vi "Object_Editor_ConfigFP.vi"(0 "reference in":refnum<class "Object_Editor.lvclass">, 5 "error in (no error)":errorcluster) -> (14 "reference out":refnum<class "Object_Editor.lvclass">, 19 "error out":errorcluster)   [LabVIEW 2022 SP3, in "Object_Editor.lvlib" / "Object_Editor.lvclass"]
uses:
  Object_Editor.lvclass
  protected/Config.ctl
  Components/ViPER.lvlibp/ViPER.lvclass
  C:/Projects/Medulla/ViPER/ViPER_ProjectTemplates/ProjectTemplates/Source/Core/ViPER/Components/ViPER.lvlibp/ViPER.lvclass
panel:
  in  "Config":T1
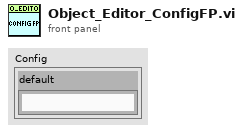
[diagram p1: front panel]
types:
  T1 = typedef "Object_Editor.lvlib/Object_Editor.lvclass/Config.ctl" = cluster{"default":string}
  T2 = enum32{"Invalid", "Standard", "Closed", "Hidden", "Minimized", "Maximized"}
  T3 = typedef "Object_Editor.lvlib/Object_Editor.lvclass/ObjectAttributes.ctl" = cluster{"Config":T1, "Tree":refnum<vi>, "Mod_Bit":bool, "File_Path":path, "Object":refnum<class "ViPER.lvclass">}
  T4 = typedef "LVRectTypeDef.ctl" = cluster{"Left":i16, "Top":i16, "Right":i16, "Bottom":i16}
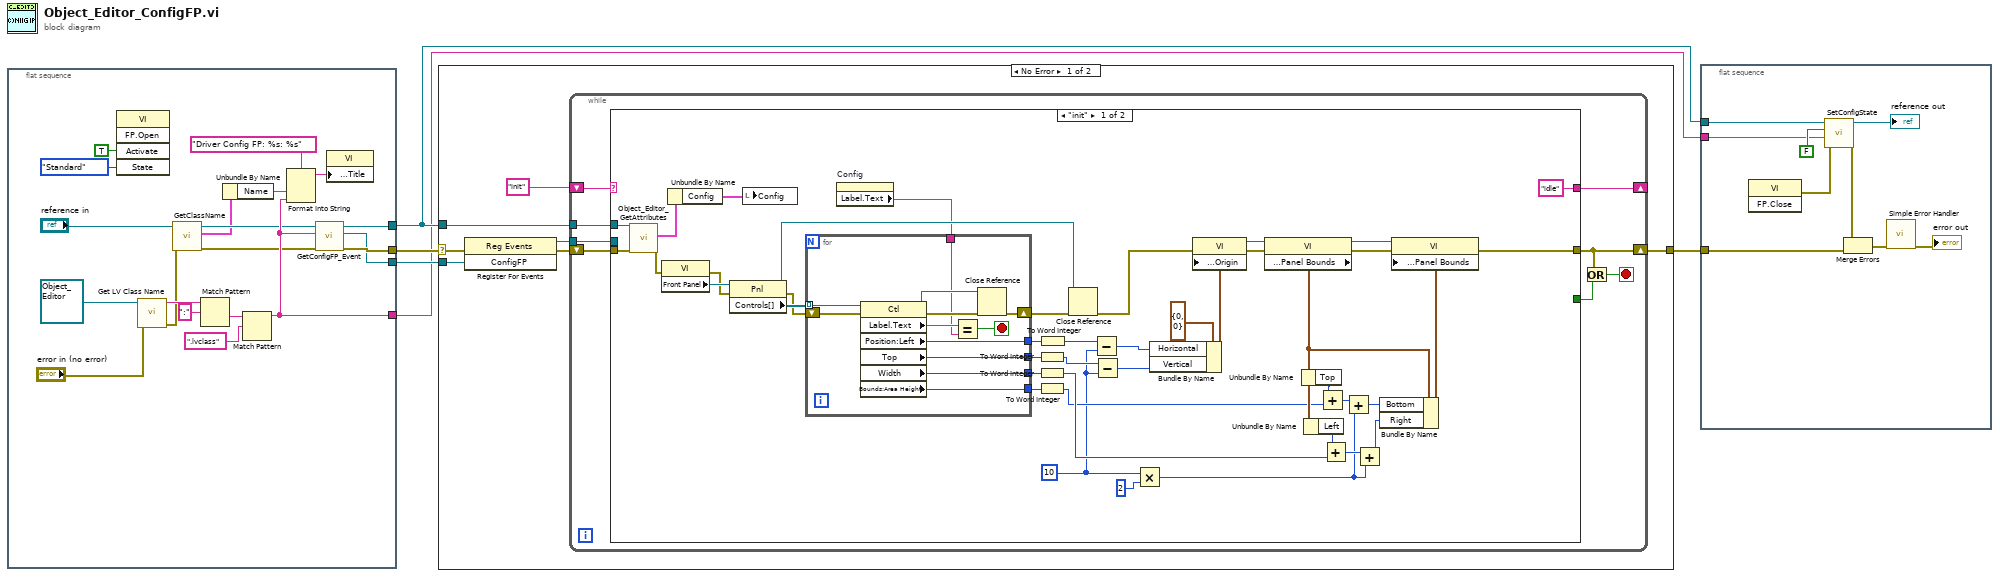
[diagram p0: block diagram]
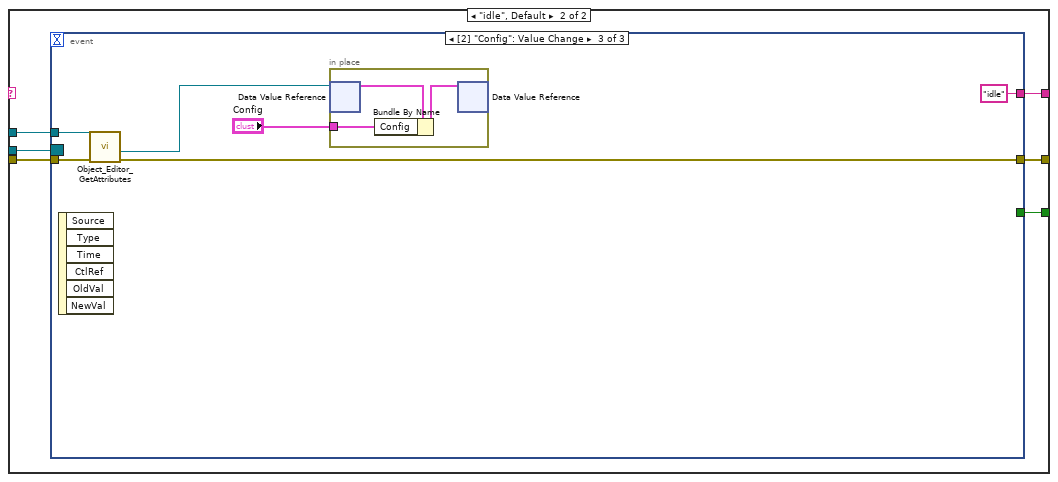
[diagram p2: hidden frame]
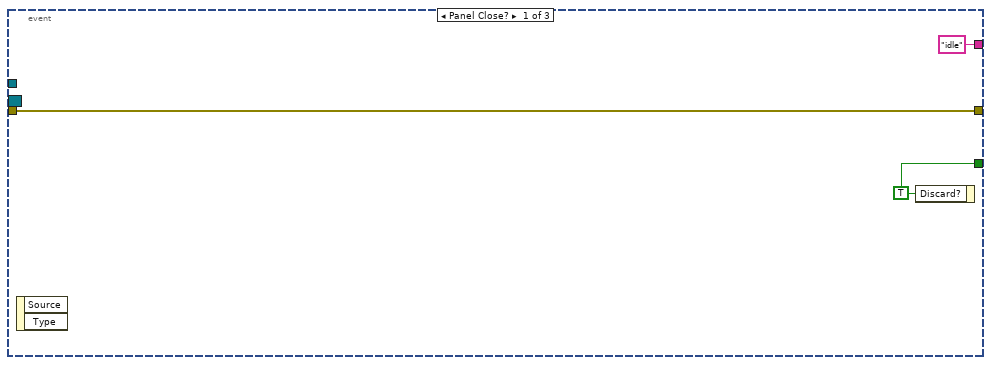
[diagram p3: hidden frame]
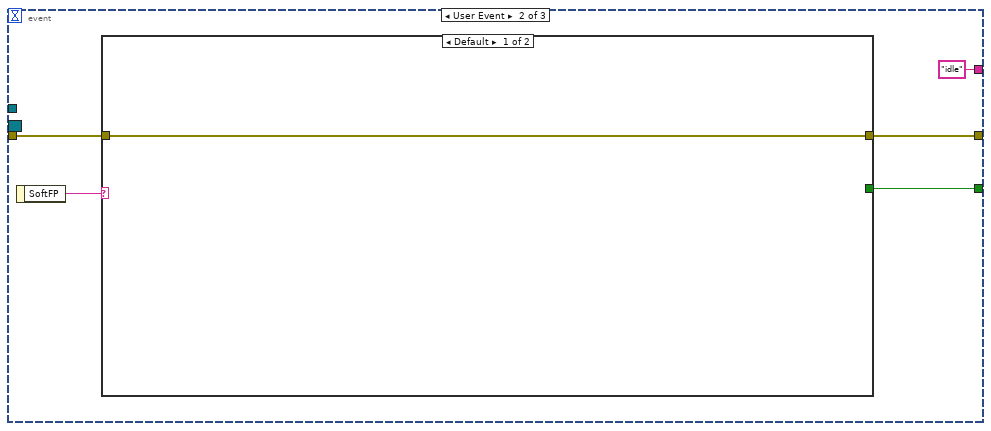
[diagram p4: hidden frame]
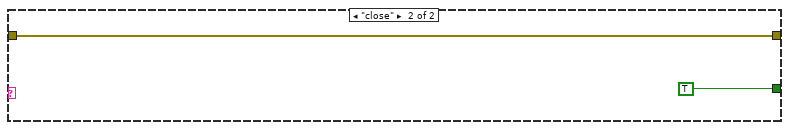
[diagram p5: hidden frame]
diagram:
  n1 = flat-sequence {
    tunnel: [w21] -> w5
    tunnel: [w22] -> w2
    tunnel: [w20] -> w3
    tunnel: [w12] -> w1
    frame #0 {
      n2 = invoke class="VI" method="FP.Open"("Activate"=TRUE ("Activate?"), "State"=T2."Standard") -> ()  [unwired: 3 in, 5 out]
      n3 = call <vilib>:"Get LV Class Name.vi"("error in (no error)"="error in (no error)", "object"=refnum<class "Object_Editor.lvclass"> refnum ("reference")) -> ("error out"=w10:errorcluster, "class name"=w18:string)  [unwired: 8 in]
      n4 = call "GetClassName.vi"("error in (no error)"=w10, "reference in"="reference in") -> ("error out"=w9:errorcluster, "Details"=w6:cluster{"Name":string, "Class":string}, "reference out"=w7:refnum<class "Object_Editor.lvclass">)  [unwired: 7 in]
      n5 = Match Pattern(string=w18, regular expression=":") -> (after substring=w17:string)  [unwired: 1 in, 3 out]
      n6 = Unbundle By Name(w6) -> ("Name"=w23:string)
      n7 = Match Pattern(string=w17, regular expression=".lvclass") -> (before substring=w12:string)  [unwired: 1 in, 3 out]
      n8 = Format Into String(format string="Driver Config FP: %s: %s", w23, w12) -> (resulting string=w25:string)  [unwired: 2 in, 1 out]
      n9 = call-dynamic "GetConfigFP_Event.vi"("error in (no error)"=w9, "Ancestor"=w12, "reference in"=w7) -> ("error out"=w21:errorcluster, "ConfigFP"=w20:refnum<user-event>, "reference out"=w22:refnum<class "Object_Editor.lvclass">)  [unwired: 6 in]
      n10 = property class="VI"("Front Panel.Title"=w25) -> ()  [unwired: 2 in, 2 out]
    }
  }
  n11 = case shown="No Error" w5 {
    selector: w5 -> [w30 w121]
    tunnel: [w26 w121] -> w4
    tunnel: w2 -> [w27 _]
    tunnel: w3 -> [w32 _]
    frame No Error {
      n12 = register-events(error in=w30, w32) -> (reference out=w31:refnum<event-registration>, error out=w29:errorcluster)  [unwired: 1 in]
      n13 = while {
        shift-right: [w37] -> w26
        shift-left: w29 -> [w40]
        tunnel: w31 -> [w39]
        tunnel: w27 -> [w38]
        shift-right: [w33] -> _
        shift-left: "init" -> [w34]
        stop <- w36 stop-if-true
        n14 = case shown="\"init\"" w34 {
          tunnel: w40 -> [w81 w100]
          tunnel: w39 -> [_ w99]
          tunnel: w38 -> [w80 w98]
          tunnel: [w44 w97] -> w37
          tunnel: [_ w96] -> w35
          tunnel: ["idle" w95] -> w33
          frame "init" {
            w46 = i16 10 ("16bit integer")
            n15 = call "Object_Editor_GetAttributes.vi"("error in (no error)"=w81, "reference in"=w80) -> ("error out"=w45:errorcluster, "Data"=w41:T3)  [unwired: 6 in, 2 out]
            n16 = property on="Property Node" class="VI"(error in=w45) -> (error out=w76:errorcluster, "Front Panel"=w78:refnum<vi>)  [unwired: 1 in, 1 out]
            n17 = Unbundle By Name(w41) -> ("Config"=w79:T1)
            n18 = property on="Property Node" class="Pnl"(reference=w78, error in=w76) -> (reference out=w51:refnum<vi>, error out=w75:errorcluster, "Controls[]"=w77:refnum<vi>[])
            n19 = local write "Config"(w79) -> ()
            n20 = property on="Config" class="Clust (strict)"() -> ("Label.Text"=w42:string)  [unwired: 2 in, 2 out]
            n21 = for {
              tunnel: w77 -> [w94] mode=indexing
              tunnel: [w90] -> w50
              tunnel: [w89] -> w48
              tunnel: [w88] -> w47
              shift-right: [w85] -> w52
              shift-left: w75 -> [w91]
              tunnel: [w87] -> w49
              tunnel: w42 -> [w83]
              stop <- w92 stop-if-true
              n22 = property class="Ctl"(reference=w94, error in=w91) -> (reference out=w84:refnum<vi>, error out=w86:errorcluster, "Label.Text"=w93:string, "Position:Left"=w90:i32, "Top"=w87:i32, "Width"=w89:u32, "Bounds:Area Height"=w88:u32)
              n23 = Equal?(x=w93, y=w83) -> (x = y?=w92:bool)
              n24 = Close Reference(reference=w84, error in (no error)=w86) -> (error out=w85:errorcluster)
            }
            n25 = To Word Integer(number=w49) -> (16bit integer=w53:i16)
            n26 = To Word Integer(number=w48) -> (16bit integer=w56:i16)
            n27 = To Word Integer(number=w47) -> (16bit integer=w55:i16)
            n28 = To Word Integer(number=w50) -> (16bit integer=w54:i16)
            n29 = Close Reference(reference=w51, error in (no error)=w52) -> (error out=w43:errorcluster)
            n30 = Subtract(x=w54, y=w46) -> (x-y=w63:i16)
            n31 = Subtract(x=w53, y=w46) -> (x-y=w64:i16)
            n32 = Multiply(x=w46, y=i16 2) -> (x*y=w57:i16)
            n33 = Bundle By Name(cluster=cluster{"Horizontal":i16, "Vertical":i16} {"Horizontal"=0, "Vertical"=0} ("Front Panel Window:Origin"), "Horizontal"=w63, "Vertical"=w64) -> (w61:cluster{"Horizontal":i16, "Vertical":i16})
            n34 = property on="Property Node" class="VI"(error in=w43, "Front Panel Window:Origin"=w61) -> (reference out=w73:refnum<vi>, error out=w59:errorcluster)  [unwired: 1 in]
            n35 = property on="Property Node" class="VI"(reference=w73, error in=w59) -> (reference out=w74:refnum<vi>, error out=w58:errorcluster, "Front Panel Window:Panel Bounds"=w65:T4)
            n36 = Unbundle By Name(w65) -> ("Top"=w66:i16)
            n37 = Unbundle By Name(w65) -> ("Left"=w67:i16)
            n38 = Add(x=w66, y=w55) -> (x+y=w71:i16)
            n39 = Add(x=w67, y=w56) -> (x+y=w69:i16)
            n40 = Add(x=w71, y=w57) -> (x+y=w72:i16)
            n41 = Add(x=w69, y=w57) -> (x+y=w70:i16)
            n42 = Bundle By Name(cluster=w65, "Bottom"=w72, "Right"=w70) -> (w68:T4)
            n43 = property on="Property Node" class="VI"(reference=w74, error in=w58, "Front Panel Window:Panel Bounds"=w68) -> (error out=w44:errorcluster)  [unwired: 1 out]
          }
          frame "idle", Default {
            n44 = event shown="[2] \"Config\": Value Change" {
              selector: w99 -> [_ _ _]
              dyn-events: _ -> [_ _ _]
              timeout: _ -> [_ _ _]
              tunnel: w100 -> [w103 w108 w117]
              tunnel: [w103 w106 w114] -> w97
              tunnel: [w102 w105 _] -> w96
              tunnel: w98 -> [_ _ w116]
              tunnel: ["idle" "idle" "idle"] -> w95
              event Panel Close? {
                w102 = TRUE ("Discard?")
                n45 = event-data() -> ()  [unwired: 1 in, 2 out]
                n46 = event-data("Discard?"=w102) -> ()  [unwired: 1 in, 1 out]
              }
              event User Event {
                n47 = event-data() -> ("SoftFP"=w107:string)  [unwired: 1 in]
                n48 = case shown="Default" w107 {
                  tunnel: w108 -> [w109 w111]
                  tunnel: [w109 w111] -> w106
                  tunnel: [_ TRUE ("Discard?")] -> w105
                  frame Default {
                  }
                  frame "close" {
                  }
                }
              }
              event Value Change {
                n49 = event-data() -> ()  [unwired: 1 in, 6 out]
                n50 = call "Object_Editor_GetAttributes.vi"("error in (no error)"=w117, "reference in"=w116) -> ("error out"=w114:errorcluster, "DataRef"=w115:refnum<data-value>)  [unwired: 6 in, 2 out]
                n51 = in-place {
                  in-place-border: "Config" -> [w118]
                  n52 = in-place-dvr #1(w115) -> (w120:T3)  [unwired: 1 out]
                  n53 = Bundle By Name(cluster=w120, "Config"=w118) -> (w119:T3)
                  n54 = in-place-dvr #1(w119) -> ()  [unwired: 2 out]
                }
              }
            }
          }
        }
        n55 = Or(x=w37, y=w35) -> (x .or. y?=w36:bool)
      }
    }
    frame Error {
    }
  }
  n56 = flat-sequence {
    tunnel: w4 -> [w128]
    tunnel: w2 -> [w125]
    tunnel: w1 -> [w123]
    frame #0 {
      n57 = invoke class="VI" method="FP.Close"() -> (error out=w127:errorcluster)  [unwired: 3 in, 2 out]
      n58 = call "SetConfigState.vi"("error in (no error)"=w127, "Ancestor"=w123, "Config Open"=FALSE ("SP Open"), "reference in"=w125) -> ("error out"=w126:errorcluster, "reference out"=→"reference out":refnum<class "Object_Editor.lvclass">)  [unwired: 6 in]
      n59 = Merge Errors(w126, w128) -> (w130:errorcluster)
      n60 = call <vilib>:"Simple Error Handler.vi"("error in (no error)"=w130) -> ("error out"=→"error out":errorcluster)  [unwired: 4 in, 4 out]
    }
  }
